vi "Out_S7F27.vi"(8 "error in (no error)":errorcluster, 10 "S7F27":T1, 11 "S7 Message Class in":refnum<class "S7 Message Class.lvclass">) -> (0 "error out":errorcluster, 3 "S7 Message Class out":refnum<class "S7 Message Class.lvclass">)   [LabVIEW 2020, in "SECS Communication.lvlib" / "S7 Message Class.lvclass"]
uses:
  S7 Message Class.lvclass
  D:/Dropbox/SECS/LabVIEW Code/Com/SECS Communication/SECS-II Class/SECS-II Class.lvclass
  S7F27.ctl
  SECS-II Class/Data Message_List.vi
  SECS-II Class/Data Message_ASCII.vi
  SECS-II Class/Data Message_U4.vi
  S7 Message Class.lvclass/S7 Message Class.ctl
  SECS-II Class/SECS-II Class.lvclass
  D:/Dropbox/SECS/LabVIEW Code/Com/SECS Communication/S7 Message Class/S7 Message Class.lvclass
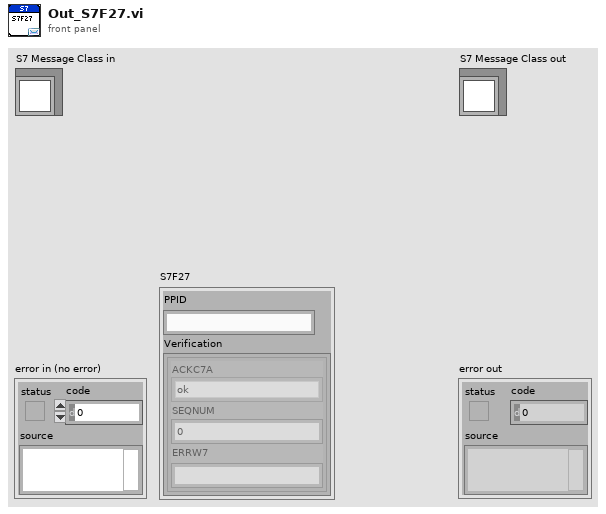
[diagram p1: front panel]
types:
  T1 = typedef "SECS Communication.lvlib/S7 Message Class.lvclass/S7F27.ctl" = cluster{"PPID":string, "Verification":cluster{"ACKC7A":enum32{"ok", "inconsistent MDLN", "inconsistent SOFTREV", "invalid CCODE", "invalid PPARM value", "error described by ERRW7"}, "SEQNUM":u32, "ERRW7":string}[]}
  T2 = cluster{"ACKC7A":enum32{"ok", "inconsistent MDLN", "inconsistent SOFTREV", "invalid CCODE", "invalid PPARM value", "error described by ERRW7"}, "SEQNUM":u32, "ERRW7":string}[]
  T3 = enum32{"ok", "inconsistent MDLN", "inconsistent SOFTREV", "invalid CCODE", "invalid PPARM value", "error described by ERRW7"}
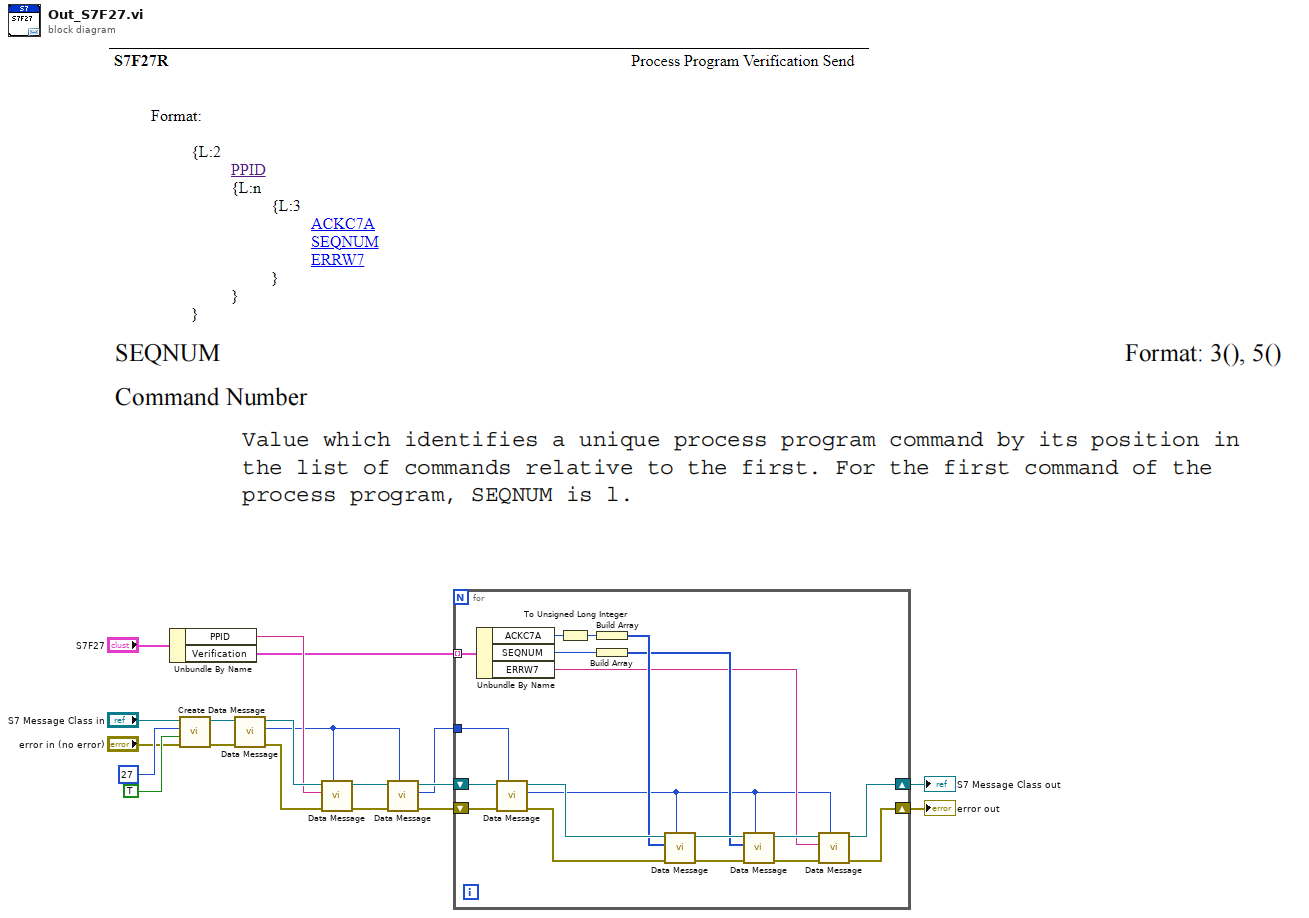
[diagram p0: block diagram]
diagram:
  n1 = Unbundle By Name("S7F27") -> ("PPID"=w10:string, "Verification"=w6:T2)
  n2 = call "Create Data Message.vi"("error in (no error)"="error in (no error)", "W-Bit"=TRUE, "Function"=u8 27, "SECS-II Class in"="S7 Message Class in") -> ("error out"=w14:errorcluster, "SECS-II Class out"=w15:refnum<class "S7 Message Class.lvclass">)  [unwired: 6 in]
  n3 = call-poly "Data Message.vi"("error in"=w14, "SECS-II Class in"=w15) -> ("error out"=w13:errorcluster, "Index"=w7:i32, "SECS-II Class out"=w12:refnum<class "S7 Message Class.lvclass">)  [unwired: 7 in]
  n4 = call-poly "Data Message.vi"("Parent Index"=w7, "error in"=w13, "Data"=w10, "SECS-II Class in"=w12) -> ("error out"=w8:errorcluster, "SECS-II Class out"=w9:refnum<class "S7 Message Class.lvclass">)  [unwired: 6 in]
  n5 = call-poly "Data Message.vi"("Parent Index"=w7, "error in"=w8, "SECS-II Class in"=w9) -> ("error out"=w5:errorcluster, "Index"=w3:i32, "SECS-II Class out"=w4:refnum<class "S7 Message Class.lvclass">)  [unwired: 6 in]
  n6 = for {
    tunnel: w6 -> [w38] mode=indexing
    shift-right: [w20] -> w1
    shift-left: w5 -> [w37]
    shift-right: [w21] -> w2
    shift-left: w4 -> [w36]
    tunnel: w3 -> [w35]
    n7 = Unbundle By Name(w38) -> ("ACKC7A"=w30:T3, "SEQNUM"=w32:u32, "ERRW7"=w23:string)
    n8 = call-poly "Data Message.vi"("Parent Index"=w35, "error in"=w37, "SECS-II Class in"=w36) -> ("error out"=w34:errorcluster, "Index"=w22:i32, "SECS-II Class out"=w33:refnum<class "S7 Message Class.lvclass">)  [unwired: 6 in]
    n9 = To Unsigned Long Integer(number=w30) -> (unsigned 32bit integer=w29:u32)
    n10 = Build Array(w29) -> (w31:u32[])
    n11 = Build Array(w32) -> (w26:u32[])
    n12 = call-poly "Data Message.vi"("Parent Index"=w22, "error in"=w34, "Data"=w31, "SECS-II Class in"=w33) -> ("error out"=w27:errorcluster, "SECS-II Class out"=w28:refnum<class "S7 Message Class.lvclass">)  [unwired: 6 in]
    n13 = call-poly "Data Message.vi"("Parent Index"=w22, "error in"=w27, "Data"=w26, "SECS-II Class in"=w28) -> ("error out"=w24:errorcluster, "SECS-II Class out"=w25:refnum<class "S7 Message Class.lvclass">)  [unwired: 6 in]
    n14 = call-poly "Data Message.vi"("Parent Index"=w22, "error in"=w24, "Data"=w23, "SECS-II Class in"=w25) -> ("error out"=w20:errorcluster, "SECS-II Class out"=w21:refnum<class "S7 Message Class.lvclass">)  [unwired: 6 in]
  }
  "error out" <- w1
  "S7 Message Class out" <- w2
